vi "Problem 11.vi"(11 "Number Grid":string="08 02 22 97 38 15 00 40 00 75 04 05 07 78 52 12 50 77 91 08\n49 49 99 40 17 81 18 57 60 87 17 40 98 43 69 48 04 56 62 00\n81 49 31 73 55 79 14 29 93 71 40 67 53 88 30 03 49 13 36 65\n52 70 95 23 04 60 11 42 69 24 68 56 01 32 56 71 37 02 36 91\n22 31 16 71 51 67 63 89 41 92 36 54 22 40 40 28 66 33 13 80\n24 47 32 60 99 03 45 02 44 75 33 53 78 36 84 20 35 17 12 50\n32 98 81 28 64 23 67 10 26 38 40 67 59 54 70 66 18 38 64 70\n67 26 20 68 02 62 12 20 95 63 94 39 63 08 40 91 66 49 94 21\n24 55 58 05 66 73 99 26 97 17 78 78 96 83 14 88 34 89 63 72\n21 36 23 09 75 00 76 44 20 45 35 14 00 61 33 97 34 31 33 95\n78 17 53 28 22 75 31 67 15 94 03 80 04 62 16 14 09 53 56 92\n16 39 05 42 96 35 31 47 55 58 88 24 00 17 54 24 36 29 85 57\n86 56 00 48 35 71 89 07 05 44 44 37 44 60 21 58 51 54 17 58\n19 80 81 68 05 94 47 69 28 73 92 13 86 52 17 77 04 89 55 40\n04 52 08 83 97 35 99 16 07 97 57 32 16 26 26 79 33 27 98 66\n88 36 68 87 57 62 20 72 03 46 33 67 46 55 12 32 63 93 53 69\n04 42 16 73 38 25 39 11 24 94 72 18 08 46 29 32 40 62 76 36\n20 69 36 41 72 30 23 88 34 62 99 69 82 67 59 85 74 04 36 16\n20 73 35 29 78 31 90 01 74 31 49 71 48 86 81 16 23 57 05 54\n01 70 54 71 83 51 54 69 16 92 33 48 61 43 52 01 89 19 67 48") -> (3 "Greatest Product":u32)   [LabVIEW 2013, in "Problem 11.lvlib"]
uses:
  Problem 11.lvlib
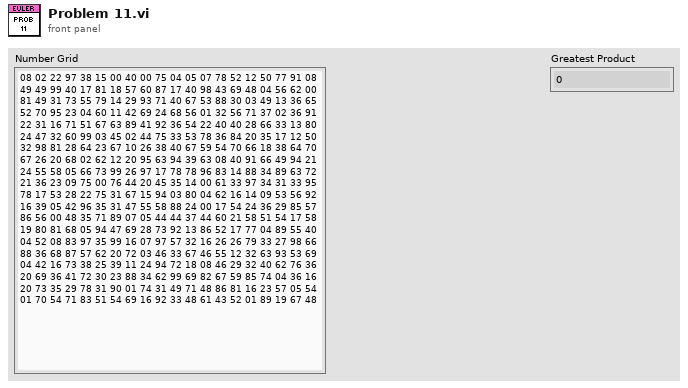
[diagram p1: front panel]
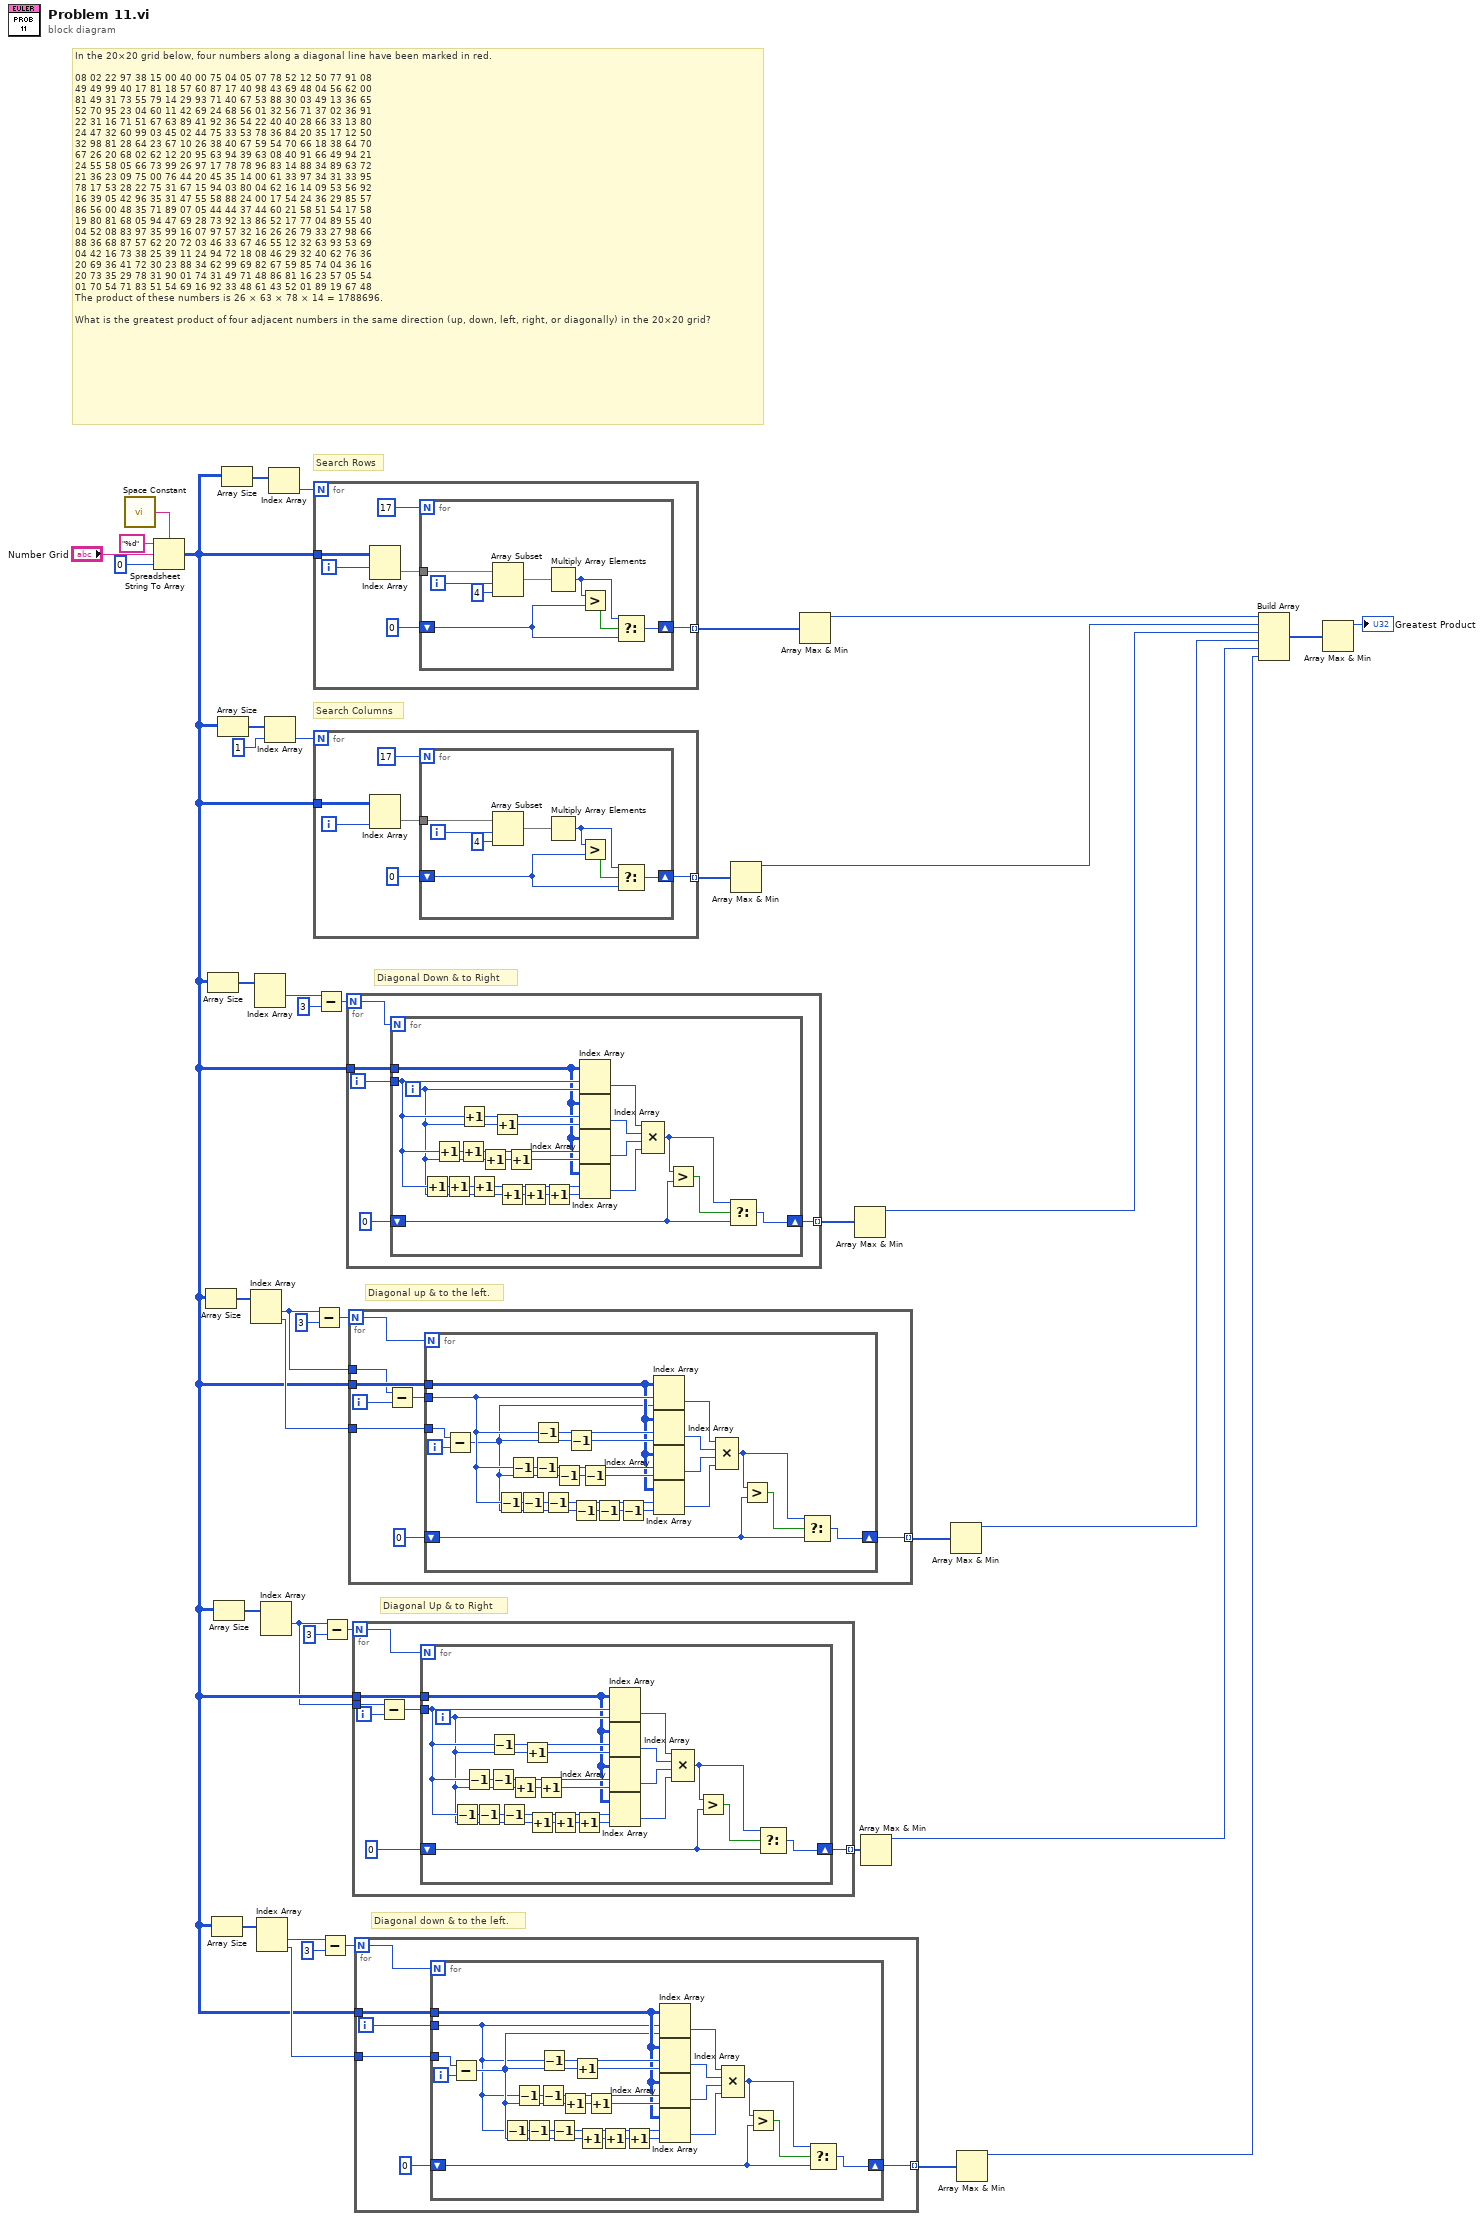
[diagram p0: block diagram]
diagram:
  # "Diagonal down & to the left."
  # "Diagonal Up & to Right"
  # "Diagonal up & to the left."
  # "Diagonal Down & to Right"
  # "Search Columns"
  # "Search Rows"
  # "In the 20×20 grid below, four numbers along a diagonal line have been marked in red.\n\n08 02 22 97 38 15 00 40 00 75 04 05 07 78 52 12 50 77 91 08\n49 49 99 40 17 81 18 57 60 87 17 40 98 43 69 48 04 56 62 00\n81 49 31 73 55 79 14 29 93 71 40 67 53 88 30 03 49 13 36 65\n52 70 95 23 04 60 11 42 69 24 68 56 01 32 56 71 37 02 36 91\n22 31 16 71 51 67 63 89 41 92 36 54 22 40 40 28 66 33 13 80\n24 47 32 60 99 03 45 02 44 75 33 53 78 36 84 20 35 17 12 50\n32 98 81 28 64 23 67 10 26 38 40 67 59 54 70 66 18 38 64 70\n67 26 20 68 02 62 12 20 95 63 94 39 63 08 40 91 66 49 94 21\n24 55 58 05 66 73 99 26 97 17 78 78 96 83 14 88 34 89 63 72\n21 36 23 09 75 00 76 44 20 45 35 14 00 61 33 97 34 31 33 95\n78 17 53 28 22 75 31 67 15 94 03 80 04 62 16 14 09 53 56 92\n16 39 05 42 96 35 31 47 55 58 88 24 00 17 54 24 36 29 85 57\n86 56 00 48 35 71 89 07 05 44 44 37 44 60 21 58 51 54 17 58\n19 80 81 68 05 94 47 69 28 73 92 13 86 52 17 77 04 89 55 40\n04 52 08 83 97 35 99 16 07 97 57 32 16 26 26 79 33 27 98 66\n88 36 68 87 57 62 20 72 03 46 33 67 46 55 12 32 63 93 53 69\n04 42 16 73 38 25 39 11 24 94 72 18 08 46 29 32 40 62 76 36\n20 69 36 41 72 30 23 88 34 62 99 69 82 67 59 85 74 04 36 16\n20 73 35 29 78 31 90 01 74 31 49 71 48 86 81 16 23 57 05 54\n01 70 54 71 83 51 54 69 16 92 33 48 61 43 52 01 89 19 67 48\nThe product of these numbers is 26 × 63 × 78 × 14 = 1788696.\n\nWhat is the greatest product of four adjacent numbers in the same direction (up, down, left, right, or diagonally) in the 20×20 grid?"
  n1 = call <vilib>:"Space Constant.vi"() -> ("String"=w40:string)
  n2 = Spreadsheet String To Array(delimiter (Tab)=w40, format string="%d", spreadsheet string="Number Grid", array type (2D Dbl)=u32 0) -> (array=w4:u32[][])
  n3 = Array Size(array=w4) -> (size(s)=w28:i32[])
  n4 = Array Size(array=w4) -> (size(s)=w33:i32[])
  n5 = Array Size(array=w4) -> (size(s)=w9:i32[])
  n6 = Array Size(array=w4) -> (size(s)=w5:i32[])
  n7 = Array Size(array=w4) -> (size(s)=w36:i32[])
  n8 = Array Size(array=w4) -> (size(s)=w38:i32[])
  n9 = Index Array(array=w28) -> (element #1=w26:i32, element #2=w25:i32)  [unwired: 2 in]
  n10 = Index Array(array=w33) -> (element #1=w32:i32)  [unwired: 2 in, 1 out]
  n11 = Index Array(array=w9) -> (element #1=w11:i32, element #2=w12:i32)  [unwired: 2 in]
  n12 = Index Array(array=w5) -> (element #1=w3:i32)  [unwired: 2 in, 1 out]
  n13 = Index Array(array=w36, index=1) -> (element=w34:i32)
  n14 = Index Array(array=w38) -> (element=w37:i32)  [unwired: 1 in]
  n15 = for {
    N: w37 -> [_]
    tunnel: w4 -> [w48]
    tunnel: [w43] -> w24 mode=indexing
    i -> [w47]
    n16 = Index Array(array=w48, index (row)=w47) -> (element=w46:u32[])  [unwired: 1 in]
    n17 = for {
      N: 17 -> [_]
      tunnel: w46 -> [w56]
      shift-right: [w52] -> w43
      shift-left: u32 0 -> [w50]
      i -> [w55]
      n18 = Array Subset(array=w56, index=w55, length=4) -> (w53:u32[])
      n19 = Multiply Array Elements(1:w53) -> (0:w51:u32)
      n20 = Greater?(x=w51, y=w50) -> (0:w49:bool)
      n21 = Select(t=w51, s=w49, f=w50) -> (s? t:f=w52:u32)
    }
  }
  n22 = for {
    N: w34 -> [_]
    tunnel: w4 -> [w62]
    tunnel: [w58] -> w23 mode=indexing
    i -> [w57]
    n23 = Index Array(array=w62, index (col)=w57) -> (element=w61:u32[])  [unwired: 1 in]
    n24 = for {
      N: 17 -> [_]
      tunnel: w61 -> [w70]
      shift-right: [w66] -> w58
      shift-left: u32 0 -> [w64]
      i -> [w69]
      n25 = Array Subset(array=w70, index=w69, length=4) -> (w67:u32[])
      n26 = Multiply Array Elements(1:w67) -> (0:w65:u32)
      n27 = Greater?(x=w65, y=w64) -> (0:w63:bool)
      n28 = Select(t=w65, s=w63, f=w64) -> (s? t:f=w66:u32)
    }
  }
  n29 = Subtract(x=w26, y=3) -> (x-y=w27:i32)
  n30 = Subtract(x=w32, y=3) -> (x-y=w31:i32)
  n31 = Subtract(x=w11, y=3) -> (x-y=w10:i32)
  n32 = Subtract(x=w3, y=3) -> (x-y=w6:i32)
  n33 = for {
    N: w31 -> [w74]
    tunnel: w4 -> [w75]
    tunnel: [w71] -> w22 mode=indexing
    i -> [w73]
    n34 = for {
      N: w74 -> [_]
      tunnel: w75 -> [w80]
      tunnel: w73 -> [w98]
      shift-right: [w76] -> w71
      shift-left: u32 0 -> [w77]
      i -> [w97]
      n35 = Increment(x=w98) -> (x+1=w90:i32)
      n36 = Increment(x=w98) -> (x+1=w94:i32)
      n37 = Increment(x=w90) -> (x+1=w89:i32)
      n38 = Increment(x=w94) -> (x+1=w93:i32)
      n39 = Increment(x=w98) -> (x+1=w96:i32)
      n40 = Increment(x=w89) -> (x+1=w88:i32)
      n41 = Increment(x=w97) -> (x+1=w92:i32)
      n42 = Increment(x=w97) -> (x+1=w95:i32)
      n43 = Increment(x=w97) -> (x+1=w87:i32)
      n44 = Increment(x=w92) -> (x+1=w91:i32)
      n45 = Increment(x=w87) -> (x+1=w86:i32)
      n46 = Increment(x=w86) -> (x+1=w85:i32)
      n47 = Index Array(array=w80, index (row)=w98, index (col)=w97) -> (element=w84:u32)
      n48 = Index Array(array=w80, index (row)=w96, index (col)=w95) -> (element=w81:u32)
      n49 = Index Array(array=w80, index (row)=w93, index (col)=w91) -> (element=w82:u32)
      n50 = Index Array(array=w80, index (row)=w88, index (col)=w85) -> (element=w83:u32)
      n51 = Compound Arithmetic op=MULTIPLY(w84, w81, w82, w83) -> (w78:u32)
      n52 = Greater?(x=w78, y=w77) -> (0:w79:bool)
      n53 = Select(t=w78, s=w79, f=w77) -> (s? t:f=w76:u32)
    }
  }
  n54 = for {
    N: w27 -> [w105]
    tunnel: w4 -> [w106]
    tunnel: [w103] -> w21 mode=indexing
    tunnel: w26 -> [w102]
    tunnel: w25 -> [w99]
    i -> [w101]
    n55 = Subtract(x=w102, y=w101) -> (x-y=w100:i32)
    n56 = for {
      N: w105 -> [_]
      tunnel: w106 -> [w114]
      tunnel: w100 -> [w131]
      shift-right: [w110] -> w103
      shift-left: u32 0 -> [w111]
      tunnel: w99 -> [w109]
      i -> [w108]
      n57 = Subtract(x=w109, y=w108) -> (x-y=w107:i32)
      n58 = Decrement(x=w131) -> (x-1=w124:i32)
      n59 = Decrement(x=w131) -> (x-1=w128:i32)
      n60 = Decrement(x=w124) -> (x-1=w123:i32)
      n61 = Decrement(x=w128) -> (x-1=w127:i32)
      n62 = Decrement(x=w131) -> (x-1=w130:i32)
      n63 = Decrement(x=w123) -> (x-1=w122:i32)
      n64 = Decrement(x=w107) -> (x-1=w126:i32)
      n65 = Decrement(x=w107) -> (x-1=w129:i32)
      n66 = Decrement(x=w107) -> (x-1=w121:i32)
      n67 = Decrement(x=w126) -> (x-1=w125:i32)
      n68 = Decrement(x=w121) -> (x-1=w120:i32)
      n69 = Decrement(x=w120) -> (x-1=w119:i32)
      n70 = Index Array(array=w114, index (row)=w131, index (col)=w107) -> (element=w118:u32)
      n71 = Index Array(array=w114, index (row)=w130, index (col)=w129) -> (element=w115:u32)
      n72 = Index Array(array=w114, index (row)=w127, index (col)=w125) -> (element=w116:u32)
      n73 = Index Array(array=w114, index (row)=w122, index (col)=w119) -> (element=w117:u32)
      n74 = Compound Arithmetic op=MULTIPLY(w118, w115, w116, w117) -> (w112:u32)
      n75 = Greater?(x=w112, y=w111) -> (0:w113:bool)
      n76 = Select(t=w112, s=w113, f=w111) -> (s? t:f=w110:u32)
    }
  }
  n77 = for {
    N: w6 -> [w137]
    tunnel: w4 -> [w138]
    tunnel: [w135] -> w13 mode=indexing
    tunnel: w3 -> [w132]
    i -> [w133]
    n78 = Subtract(x=w132, y=w133) -> (x-y=w134:i32)
    n79 = for {
      N: w137 -> [_]
      tunnel: w138 -> [w143]
      tunnel: w134 -> [w161]
      shift-right: [w139] -> w135
      shift-left: u32 0 -> [w140]
      i -> [w160]
      n80 = Decrement(x=w161) -> (x-1=w153:i32)
      n81 = Decrement(x=w161) -> (x-1=w157:i32)
      n82 = Decrement(x=w153) -> (x-1=w152:i32)
      n83 = Decrement(x=w157) -> (x-1=w156:i32)
      n84 = Decrement(x=w161) -> (x-1=w159:i32)
      n85 = Decrement(x=w152) -> (x-1=w151:i32)
      n86 = Increment(x=w160) -> (x+1=w155:i32)
      n87 = Increment(x=w160) -> (x+1=w158:i32)
      n88 = Increment(x=w160) -> (x+1=w150:i32)
      n89 = Increment(x=w155) -> (x+1=w154:i32)
      n90 = Increment(x=w150) -> (x+1=w149:i32)
      n91 = Increment(x=w149) -> (x+1=w148:i32)
      n92 = Index Array(array=w143, index (row)=w161, index (col)=w160) -> (element=w147:u32)
      n93 = Index Array(array=w143, index (row)=w159, index (col)=w158) -> (element=w144:u32)
      n94 = Index Array(array=w143, index (row)=w156, index (col)=w154) -> (element=w145:u32)
      n95 = Index Array(array=w143, index (row)=w151, index (col)=w148) -> (element=w146:u32)
      n96 = Compound Arithmetic op=MULTIPLY(w147, w144, w145, w146) -> (w141:u32)
      n97 = Greater?(x=w141, y=w140) -> (0:w142:bool)
      n98 = Select(t=w141, s=w142, f=w140) -> (s? t:f=w139:u32)
    }
  }
  n99 = for {
    N: w10 -> [w166]
    tunnel: w4 -> [w167]
    tunnel: [w164] -> w14 mode=indexing
    tunnel: w12 -> [w163]
    i -> [w162]
    n100 = for {
      N: w166 -> [_]
      tunnel: w167 -> [w176]
      shift-right: [w172] -> w164
      shift-left: u32 0 -> [w173]
      tunnel: w163 -> [w171]
      tunnel: w162 -> [w168]
      i -> [w170]
      n101 = Subtract(x=w171, y=w170) -> (x-y=w169:i32)
      n102 = Decrement(x=w168) -> (x-1=w186:i32)
      n103 = Decrement(x=w168) -> (x-1=w190:i32)
      n104 = Decrement(x=w186) -> (x-1=w185:i32)
      n105 = Decrement(x=w190) -> (x-1=w189:i32)
      n106 = Decrement(x=w168) -> (x-1=w192:i32)
      n107 = Decrement(x=w185) -> (x-1=w184:i32)
      n108 = Increment(x=w169) -> (x+1=w188:i32)
      n109 = Increment(x=w169) -> (x+1=w191:i32)
      n110 = Increment(x=w169) -> (x+1=w183:i32)
      n111 = Increment(x=w188) -> (x+1=w187:i32)
      n112 = Increment(x=w183) -> (x+1=w182:i32)
      n113 = Increment(x=w182) -> (x+1=w181:i32)
      n114 = Index Array(array=w176, index (row)=w168, index (col)=w169) -> (element=w180:u32)
      n115 = Index Array(array=w176, index (row)=w192, index (col)=w191) -> (element=w177:u32)
      n116 = Index Array(array=w176, index (row)=w189, index (col)=w187) -> (element=w178:u32)
      n117 = Index Array(array=w176, index (row)=w184, index (col)=w181) -> (element=w179:u32)
      n118 = Compound Arithmetic op=MULTIPLY(w180, w177, w178, w179) -> (w174:u32)
      n119 = Greater?(x=w174, y=w173) -> (0:w175:bool)
      n120 = Select(t=w174, s=w175, f=w173) -> (s? t:f=w172:u32)
    }
  }
  n121 = Array Max & Min(array=w23) -> (max value=w19:u32)  [unwired: 3 out]
  n122 = Array Max & Min(array=w24) -> (max value=w20:u32)  [unwired: 3 out]
  n123 = Array Max & Min(array=w22) -> (max value=w18:u32)  [unwired: 3 out]
  n124 = Array Max & Min(array=w13) -> (max value=w1:u32)  [unwired: 3 out]
  n125 = Array Max & Min(array=w21) -> (max value=w17:u32)  [unwired: 3 out]
  n126 = Array Max & Min(array=w14) -> (max value=w2:u32)  [unwired: 3 out]
  n127 = Build Array(w20, w19, w18, w17, w1, w2) -> (w16:u32[])
  n128 = Array Max & Min(array=w16) -> (max value=→"Greatest Product":u32)  [unwired: 3 out]
